vi "PathPlanner_EventMarker_FromJSON_Data.vi"(8 "Cmd Index":i32, 9 "Index":i32, 10 "JSON String":string, 11 "In Command Data":T2) -> (0 "error out":errorcluster, 3 "out Command Data":T2)   [LabVIEW 2019, in "PathPlanner24.lvlib"]
doc: "Internal function to parse JSON data for Event Markers. This is data that is different for each different type of Event Marker command.\n\nNotes:\n--------\nCurrently the only type of commands that can be issued are Boolean commands. The value is forced to TRUE when the command is issued.\n\nThe following table lists the actions performed for different types of commands:\n - Unknown - nothing - not supported.\n - Wait - nothing - not supported\n - Named - Issue boolean command with TRUE value using the \"name\" as the command name.\n - Path - nothing - not supported\n - Sequential, Parallel, Race, Deadline - Issue boolean command with TRUE value for each of the commands contained in the \"commands\" array. The value for \"name\" is used as the command name."
uses:
  PathPlanner24.lvlib
  ENum/PathPlanner_CommandUtil_Type_ENUM.ctl
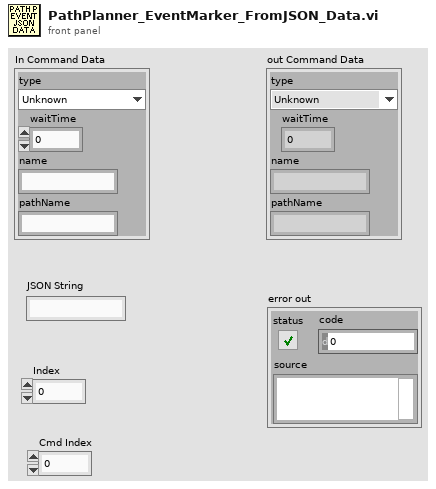
[diagram p1: front panel]
types:
  T1 = typedef "PathPlanner24.lvlib/PathPlanner_CommandUtil_Type_ENUM.ctl" = enum16{"Unknown", "Wait", "Named", "Path", "Sequential", "Parallel", "Race", "Deadline"}
  T2 = cluster{"type":T1, "waitTime":dbl, "name":string, "pathName":string}
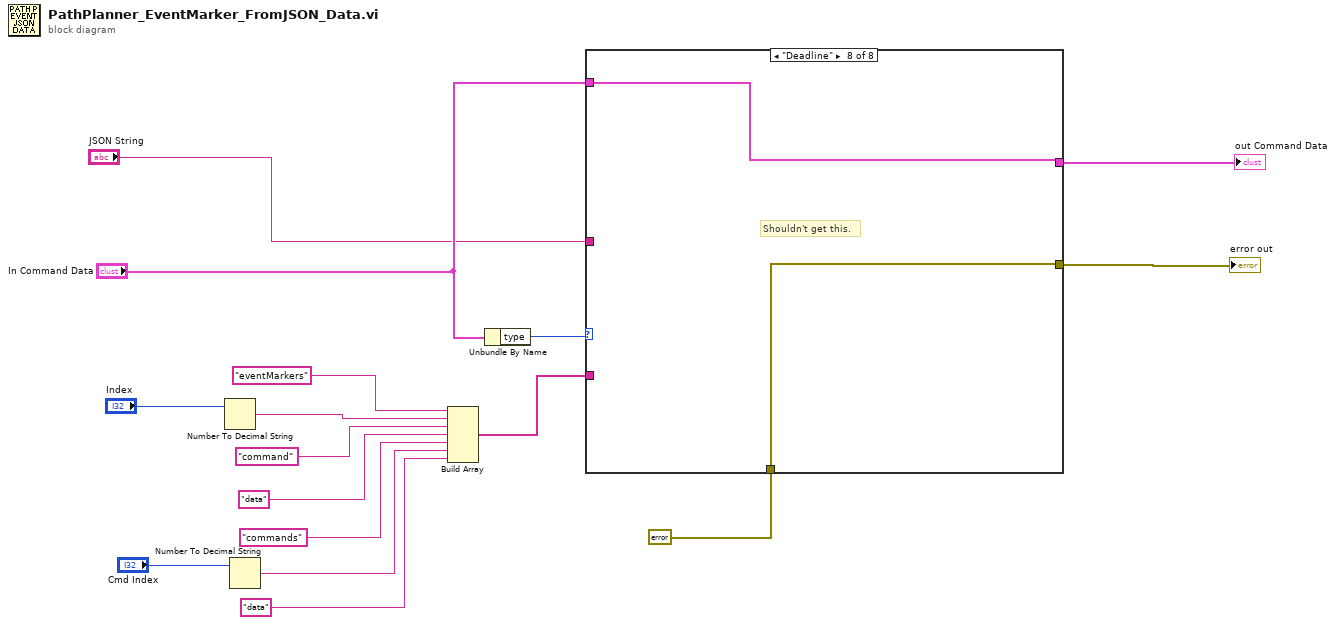
[diagram p0: block diagram]
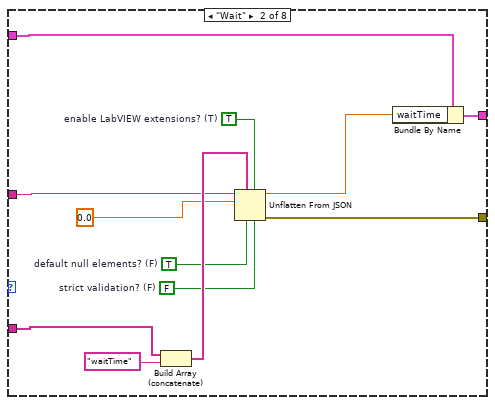
[diagram p3: hidden frame]
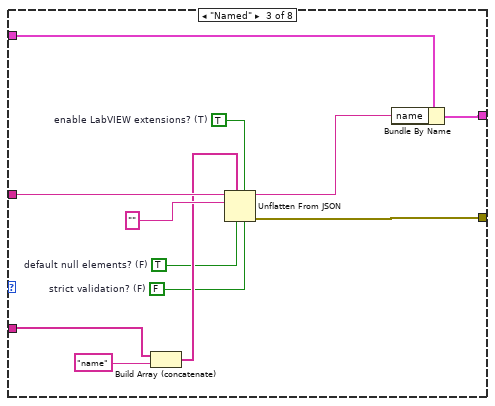
[diagram p4: hidden frame]
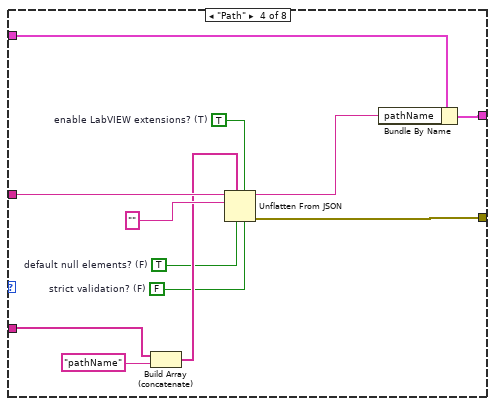
[diagram p5: hidden frame]
diagram:
  n1 = Number To Decimal String(number="Index") -> (decimal integer string=w12:string)  [unwired: 1 in]
  n2 = Number To Decimal String(number="Cmd Index") -> (decimal integer string=w8:string)  [unwired: 1 in]
  n3 = Build Array("eventMarkers", w12, "command", "data", "commands", w8, "data") -> (w4:string[])
  n4 = Unbundle By Name("In Command Data") -> ("type"=w16:T1)
  n5 = case shown="\"Deadline\"" w16 {
    tunnel: "In Command Data" -> [w18 w23 w33 w45 w56 w58 w60 w62]
    tunnel: [w18 w20 w34 w46 w56 w58 w60 w62] -> w5
    tunnel: w4 -> [_ w24 w42 w54 _ _ _ _]
    tunnel: "JSON String" -> [_ w22 w40 w52 _ _ _ _]
    tunnel: [w17 w19 w31 w43 w55 w57 w59 w61] -> w2
    tunnel: errorcluster {"status"=FALSE, "code"=0, "source"=""} ("error out") -> [w17 _ _ _ w55 w57 w59 w61]
    frame "Unknown", Default {
    }
    frame "Wait" {
      w26 = FALSE  # strict validation? (F)
      w27 = TRUE  # default null elements? (F)
      w28 = TRUE  # enable LabVIEW extensions? (T)
      n6 = Build Array (concatenate)(w24, "waitTime") -> (w29:string[])
      n7 = Unflatten From JSON(path=w29, enable LabVIEW extensions? (T)=w28, JSON string=w22, type and defaults=0.0, default null elements? (F)=w27, strict validation? (F)=w26) -> (value=w25:dbl, error out=w19:errorcluster)  [unwired: 1 in]
      n8 = Bundle By Name(cluster=w23, "waitTime"=w25) -> (w20:T2)
    }
    frame "Named" {
      w35 = FALSE  # strict validation? (F)
      w36 = TRUE  # default null elements? (F)
      w37 = TRUE  # enable LabVIEW extensions? (T)
      n9 = Build Array (concatenate)(w42, "name") -> (w38:string[])
      n10 = Unflatten From JSON(path=w38, enable LabVIEW extensions? (T)=w37, JSON string=w40, type and defaults="", default null elements? (F)=w36, strict validation? (F)=w35) -> (value=w32:string, error out=w31:errorcluster)  [unwired: 1 in]
      n11 = Bundle By Name(cluster=w33, "name"=w32) -> (w34:T2)
    }
    frame "Path" {
      w47 = FALSE  # strict validation? (F)
      w48 = TRUE  # default null elements? (F)
      w49 = TRUE  # enable LabVIEW extensions? (T)
      n12 = Build Array (concatenate)(w54, "pathName") -> (w50:string[])
      n13 = Unflatten From JSON(path=w50, enable LabVIEW extensions? (T)=w49, JSON string=w52, type and defaults="", default null elements? (F)=w48, strict validation? (F)=w47) -> (value=w44:string, error out=w43:errorcluster)  [unwired: 1 in]
      n14 = Bundle By Name(cluster=w45, "pathName"=w44) -> (w46:T2)
    }
    frame "Sequential" {
      # "shouldn't get this."
    }
    frame "Parallel" {
      # "Shouldn't get this."
    }
    frame "Race" {
      # "Shouldn't get this."
    }
    frame "Deadline" {
      # "Shouldn't get this."
    }
  }
  "out Command Data" <- w5
  "error out" <- w2
